vi "Align Buffers.vi"(8 "error in (no error)":errorcluster, 10 "Transfer Group Buffers":refnum<class "Buffers.lvclass">, 11 "Transfer in":refnum<class "Transfer.lvclass">) -> (0 "error out":errorcluster, 3 "Transfer out":refnum<class "Transfer.lvclass">)   [LabVIEW 2017, in "DSF Core.lvlib" / "Transfer.lvclass"]
uses:
  Transfer.lvclass
  Buffer/Buffers.lvclass
  Transfer.lvclass/Transfer.ctl
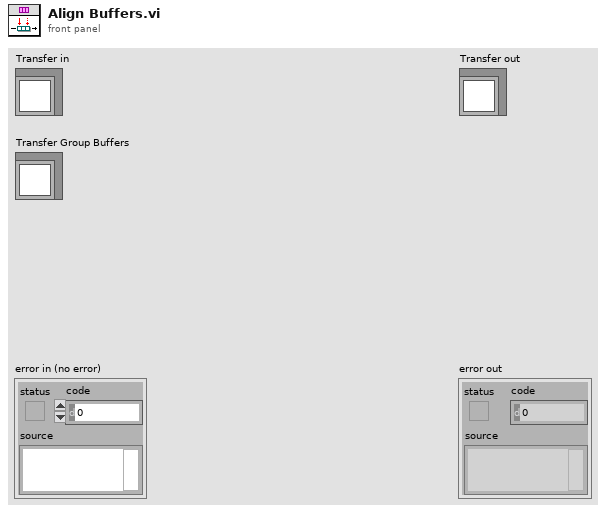
[diagram p1: front panel]
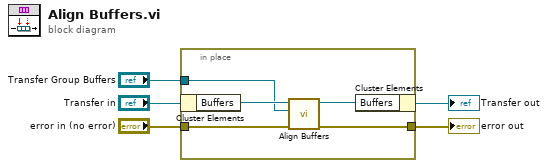
[diagram p0: block diagram]
diagram:
  n1 = in-place {
    in-place-border: "error in (no error)" -> [w9]
    in-place-border: [w8] -> w1
    in-place-border: "Transfer Group Buffers" -> [w6]
    n2 = in-place-cluster #1("Transfer in") -> ("Buffers"=w10:refnum<class "Buffers.lvclass">)
    n3 = call "Align Buffers.vi"("error in (no error)"=w9, "base Buffers"=w6, "Buffers in"=w10) -> ("error out"=w8:errorcluster, "Buffers out"=w7:refnum<class "Buffers.lvclass">)  [unwired: 7 in]
    n4 = in-place-cluster #1("Buffers"=w7) -> (→"Transfer out":refnum<class "Transfer.lvclass">)
  }
  "error out" <- w1
